vi "Power Peak Data Acquisition Sweep.vi"() -> (0 "df":dbl format="%0.2f", 1 "Power Spectrum (V^2 rms)":dbl[](array[numeric]))   [LabVIEW 2013]
uses:
  <vilib>/DAQmx/read.llb/DAQmx Read (Analog 1D DBL 1Chan NSamp).vi
  <vilib>/DAQmx/create/channels.llb/DAQmx Create Channel (AI-Voltage-Basic).vi
  <vilib>/DAQmx/configure/timing.llb/DAQmx Timing (Sample Clock).vi
  <vilib>/DAQmx/miscellaneous.llb/DAQmx Fill In Error Info.vi
  <vilib>/Analysis/NI_AALPro.lvlib
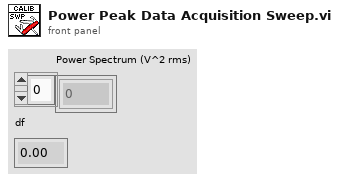
[diagram p1: front panel]
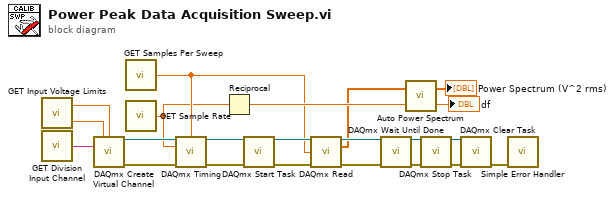
[diagram p0: block diagram]
diagram:
  n1 = call "GET Input Voltage Limits.vi"() -> ("Maximum Input Voltage"=w2:dbl, "Minimum Input Voltage"=w1:dbl)
  n2 = call "GET Division Input Channel.vi"() -> ("Division Input Channel"=w3:string)
  n3 = call-poly <vilib>:"DAQmx Create Virtual Channel.vi"("maximum value"=w2, "minimum value"=w1, "physical channels"=w3) -> ("task out"=w22:refnum<k21>, "error out"=w21:errorcluster)  [unwired: 11 in]
  n4 = call "GET Samples Per Sweep.vi"() -> ("Samples Per Sweep"=w5:dbl)
  n5 = call "GET Sample Rate.vi"() -> ("Calibration Sample Rate"=w4:dbl)
  n6 = call-poly <vilib>:"DAQmx Timing.vi"("task/channels in"=w22, "samples per channel"=w5, "rate"=w4, "error in"=w21) -> ("task out"=w20:refnum<k21>, "error out"=w19:errorcluster)  [unwired: 10 in]
  n7 = Reciprocal(x=w4) -> (1/x=w10:dbl)
  n8 = call <vilib>:"DAQmx Start Task.vi"("task/channels in"=w20, "error in"=w19) -> ("task out"=w18:refnum<k21>, "error out"=w17:errorcluster)  [unwired: 12 in]
  n9 = call-poly <vilib>:"DAQmx Read.vi"("task/channels in"=w18, "number of samples per channel"=w5, "error in"=w17) -> ("task out"=w16:refnum<k21>, "data"=w8:dbl[], "error out"=w15:errorcluster)  [unwired: 10 in]
  n10 = call <vilib>:"DAQmx Wait Until Done.vi"("task/channels in"=w16, "error in"=w15) -> ("task out"=w14:refnum<k21>, "error out"=w13:errorcluster)  [unwired: 12 in]
  n11 = call <vilib>:"Auto Power Spectrum.vi"("dt"=w10, "Signal (V)"=w8) -> ("df"=→"df":dbl, "Power Spectrum (V^2 rms)"=→"Power Spectrum (V^2 rms)":dbl[])
  n12 = call <vilib>:"DAQmx Stop Task.vi"("task/channels in"=w14, "error in"=w13) -> ("task out"=w12:refnum<k21>, "error out"=w11:errorcluster)  [unwired: 12 in]
  n13 = call <vilib>:"DAQmx Clear Task.vi"("task in"=w12, "error in"=w11) -> ("error out"=w9:errorcluster)  [unwired: 13 in]
  n14 = call <vilib>:"Simple Error Handler.vi"("error in (no error)"=w9) -> ()  [unwired: 4 in, 5 out]
